vi "10kA Tripping Test.vi"() -> ()   [LabVIEW 2009]
uses:
  Global 6KA.vi
  <vilib>/measure/mamon.llb/Waveform Peak Detection for 1 Chan.vi
  <vilib>/measure/madcrms.llb/Basic Averaged DC-RMS for 1 Chan.vi
  <vilib>/measure/NI_MAPro.lvlib
  <vilib>/Analysis/NI_AALBase.lvlib
panel:
  in  "计算方式选择":bool
  out "状态显示":string
  in  "Peak to RMS":bool
  out "calc led":bool
  out "start led":bool
  in  "Start":bool
  in  "Calculate":bool
  in  "Pulse 50A":enum32{"50A"}(tab)
  in  "50A switch":bool=TRUE
  out "power on time":dbl format="%.1f"
  out "Current":dbl format="%.2f"
  in  "I/V Tab":enum32{"设置", "电流波形显示 ", "电压波形显示"}(tab)
  in  "300V":dbl=1.0 format="%.6g"
  in  "确认":bool
  in  "Current Cal.":dbl[](array[numeric])=[1.0, 1.0, 1.0, 1.0] format="%.6f"
  in  "Save setting":bool
  in  "采样频率":u16=50
  in  "采集时间":i32=500 min=20 max=60000 step=1
  in  "预期试验电流":dbl=50.0
  in  "保存图片":bool
  out "End time":dbl
  out "Start time":dbl
  out "Current Graph":cluster{"Y":dbl[], "Y":dbl[]}[](graph)
  out "voltage graph":cluster{"Y":dbl[], "Y":dbl[]}[](graph)
  in  "Quit":bool
  in  "电流传感器量程":i8(slide)=1 min=1 max=50 step=1 scale=1.0..4.0
  # "D1.25KA 剩余电流测试装置  v1.0"
  # "1250A"
  # "300A"
  # "50A"
  # "10A"
  # "脱扣电流和脱扣时间"
  # "(A)"
  # "(ms)"
  # "手动"
  # "自动"
  # "1-50A"
  # "Other"
  # "采集参数"
  # "计量系数"
  # "10A"
  # "(k/s)"
  # "50A"
  # "300A"
  # "1250A"
  # "(ms)"
  # "(A)"
  # "长沙研诺电气设备有限公司"
  # "请将鼠标移动到界面上任意位置，停留2秒钟后会显示帮助信息!"
  # "长沙研诺电气设备有限公司"
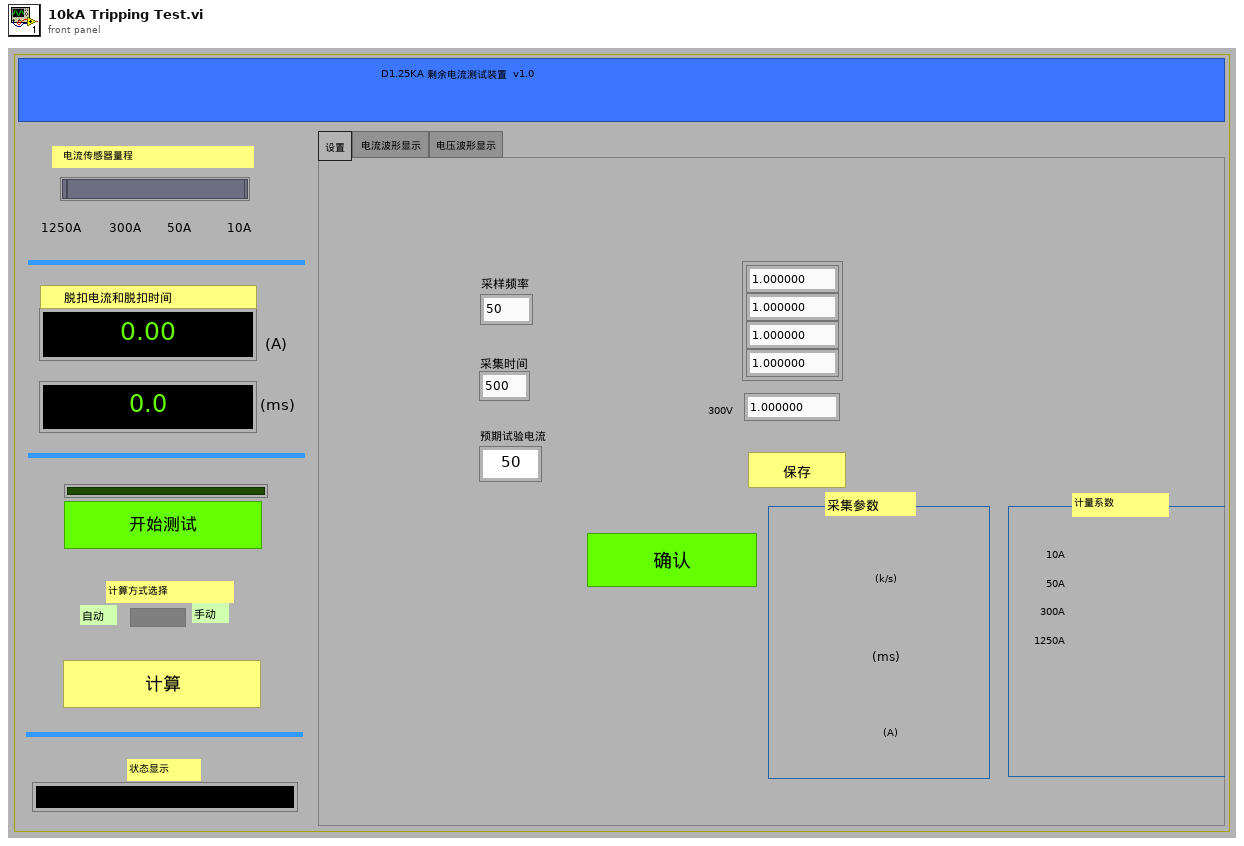
[diagram p1: front panel]
types:
  T1 = enum16{"open", "replace", "create", "open or create", "replace or create", "replace or create with confirmation"}
  T2 = typedef "LVCursorListTypeDef.ctl" = cluster{"Name":string, "Color":u32, "Style":u8, "Point Style":u8, "Name Visible":bool, "Allow Drag":bool, "Cursor Mode":u32, "Plot":i32, "Index":i32, "Position":cluster{"X":dbl, "Y":dbl}, "X Scale":u32, "Y Scale":u32, "Watch Plots":i32[], "Watch All Plots":bool, "Plot Area":i32, "Label Offset":cluster{"X":dbl, "Y":dbl}}[]
  T3 = cluster{"Name":string, "Color":u32, "Style":u8, "Point Style":u8, "Name Visible":bool, "Allow Drag":bool, "Cursor Mode":u32, "Plot":i32, "Index":i32, "Position":cluster{"X":dbl, "Y":dbl}, "X Scale":u32, "Y Scale":u32, "Watch Plots":i32[], "Watch All Plots":bool, "Plot Area":i32, "Label Offset":cluster{"X":dbl, "Y":dbl}}
  T4 = typedef "imagedata.ctl" = cluster{"image type":i32, "image depth":i32, "image":u8[], "mask":u8[], "colors":u32[], "Rectangle":cluster{"left":i16, "top":i16, "right":i16, "bottom":i16}}
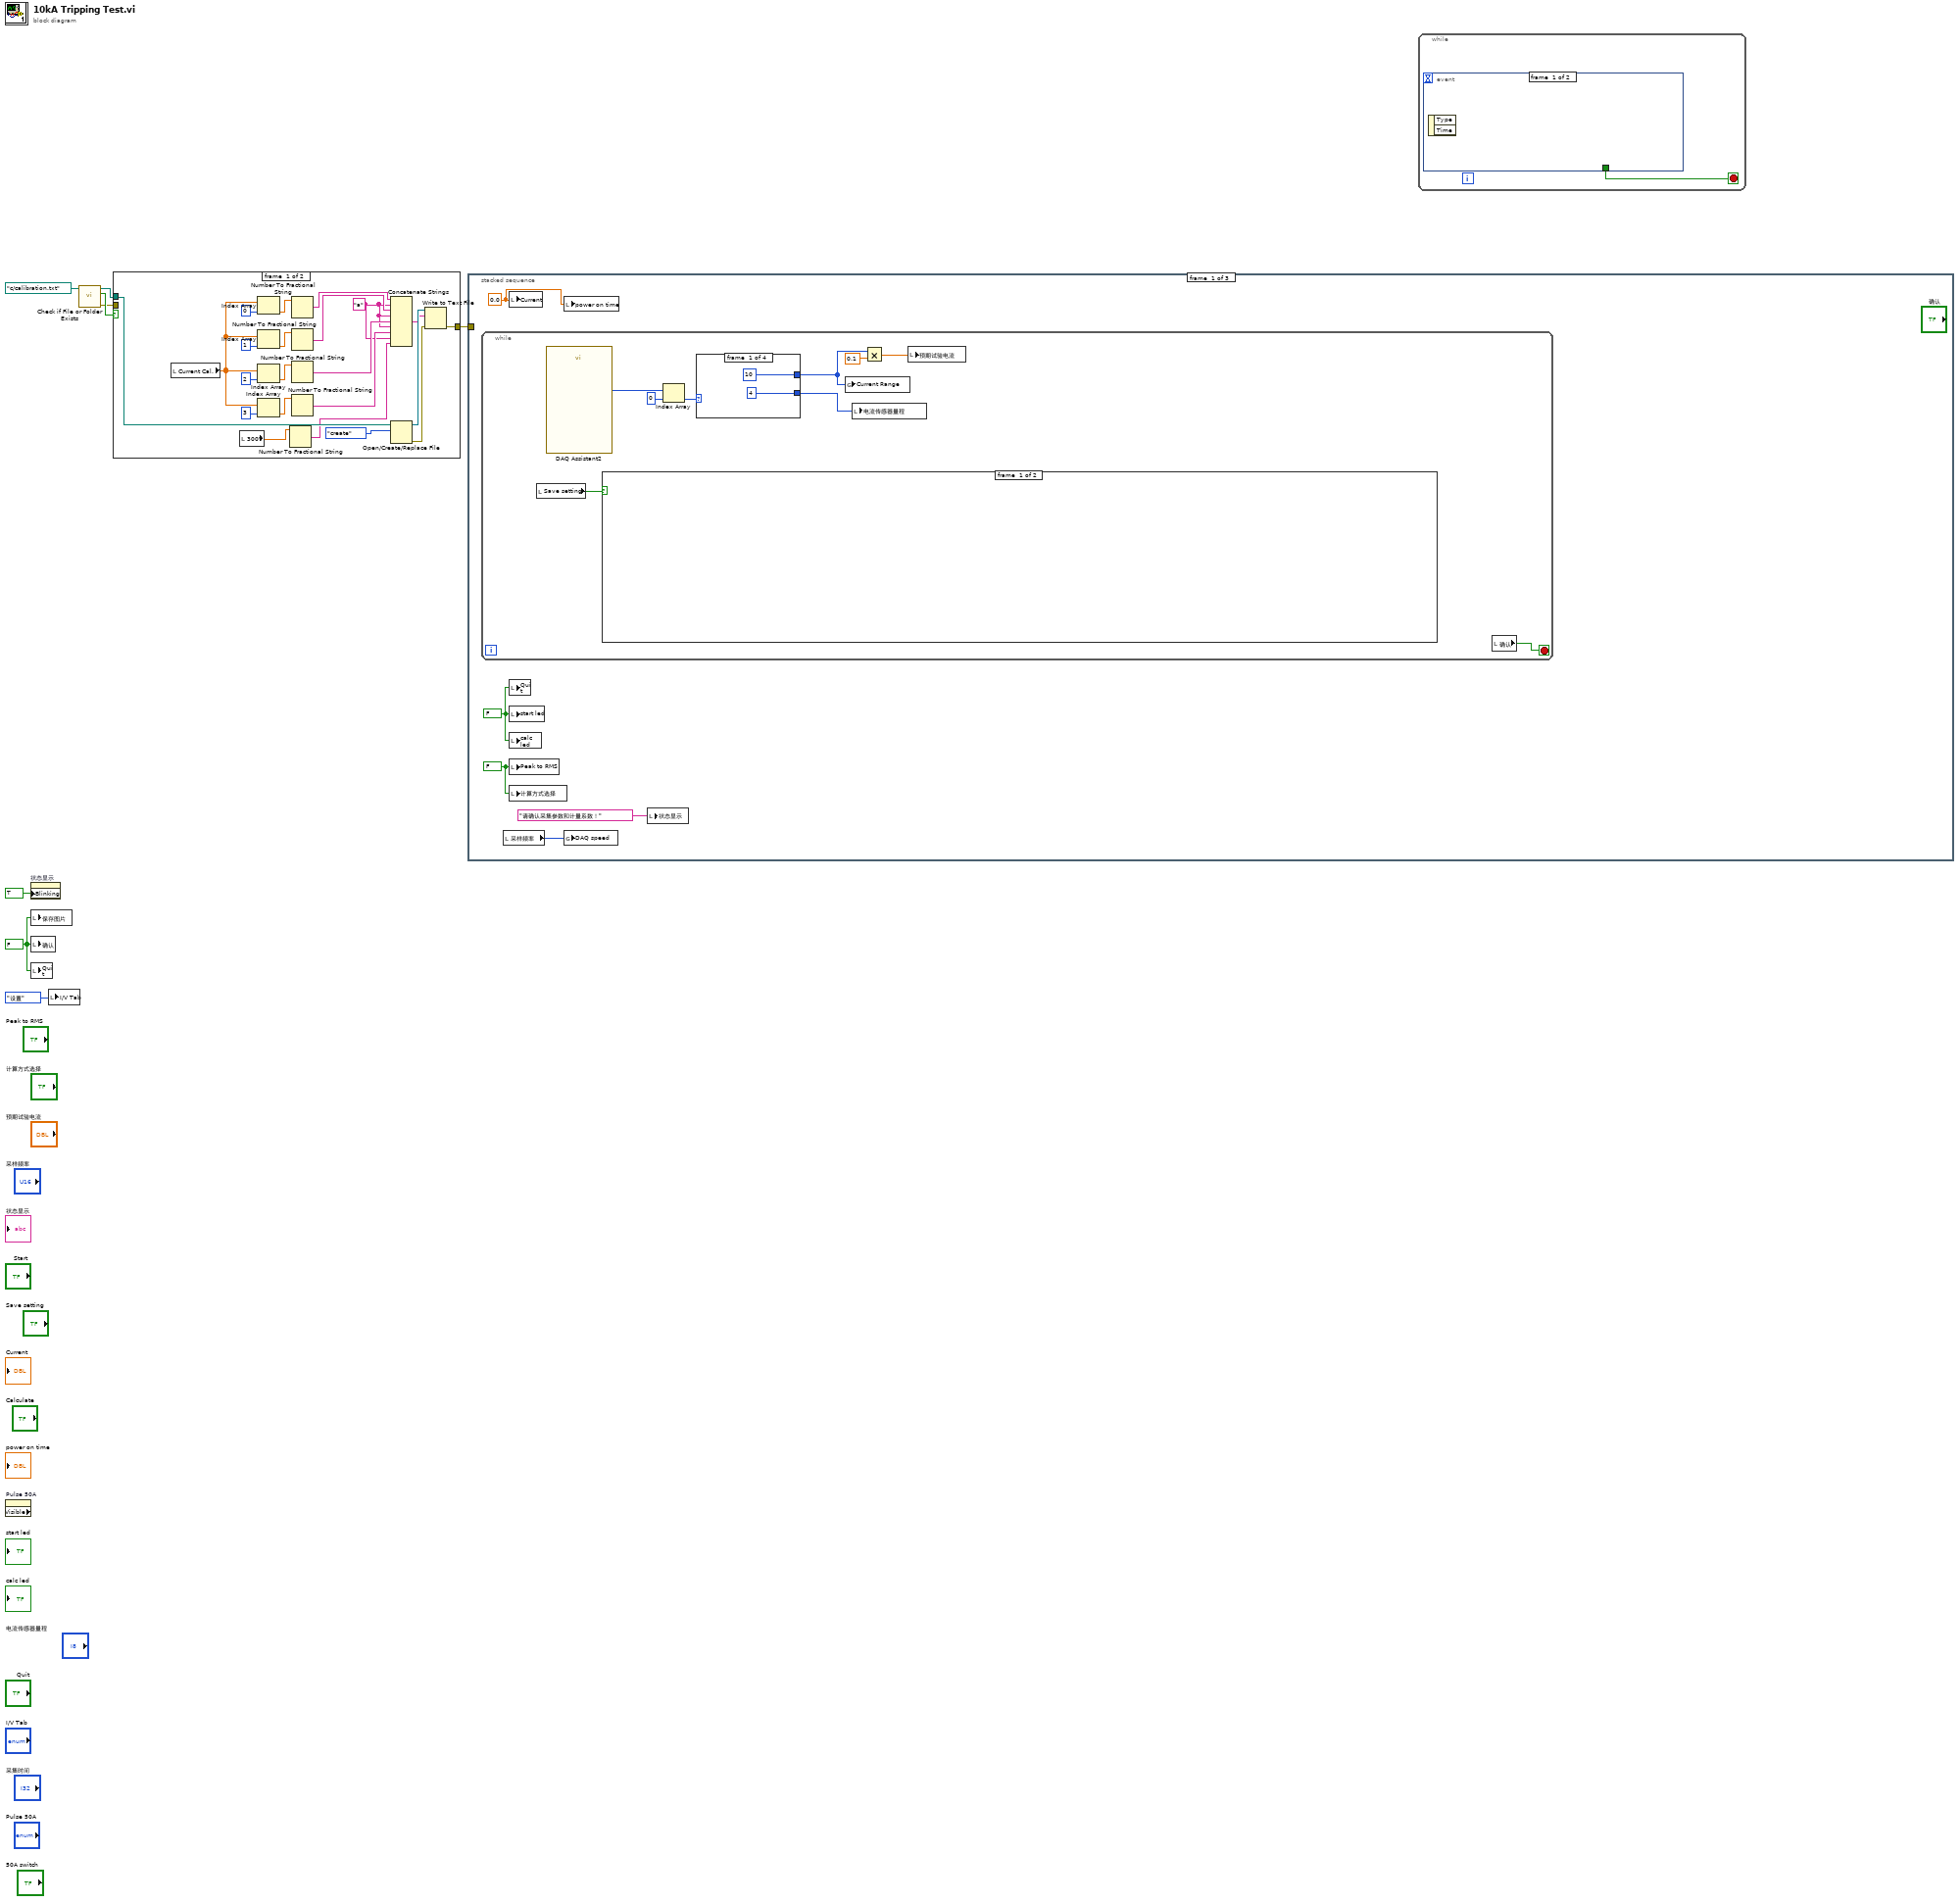
[diagram p0: block diagram]
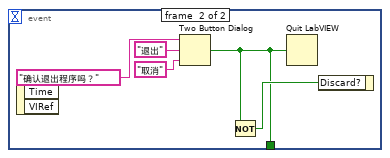
[diagram p2: hidden frame]
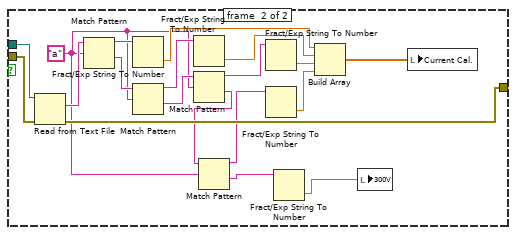
[diagram p3: hidden frame]
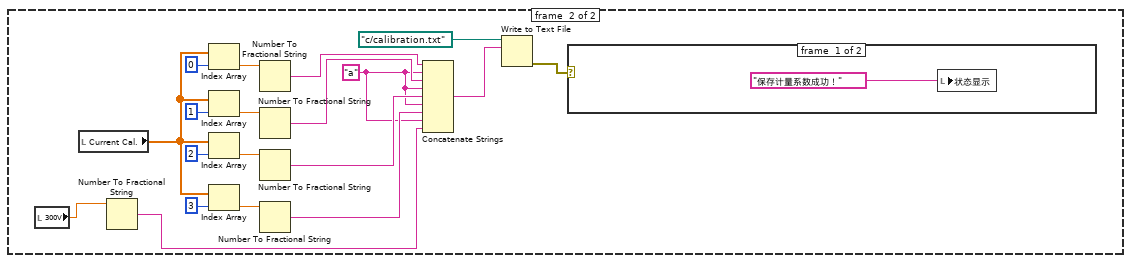
[diagram p4: hidden frame]
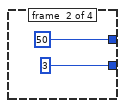
[diagram p6: hidden frame]
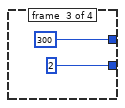
[diagram p7: hidden frame]
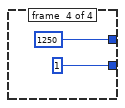
[diagram p8: hidden frame]
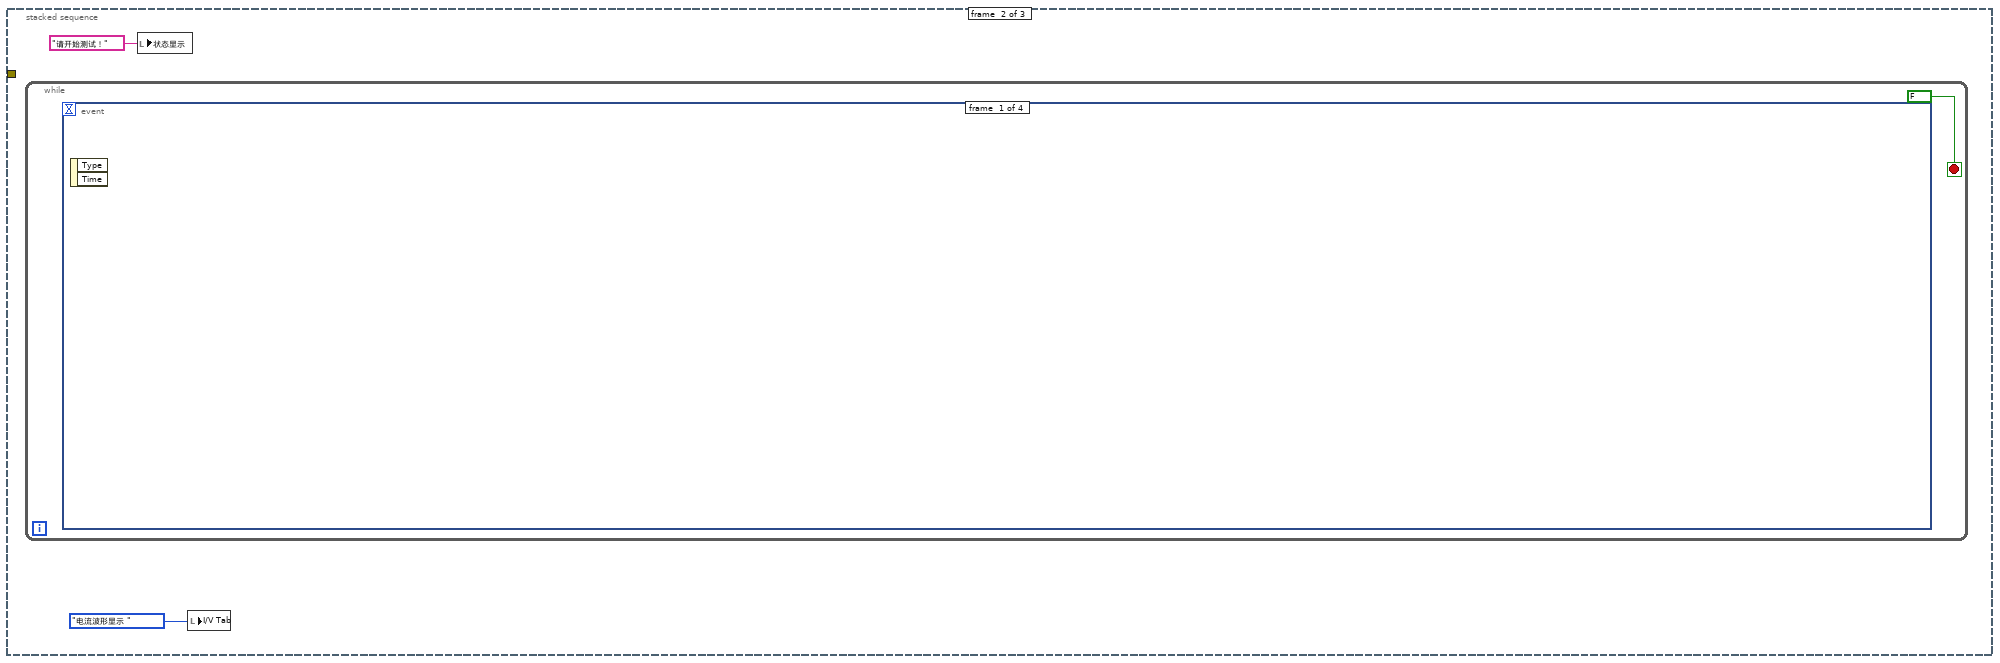
[diagram p9: hidden frame]
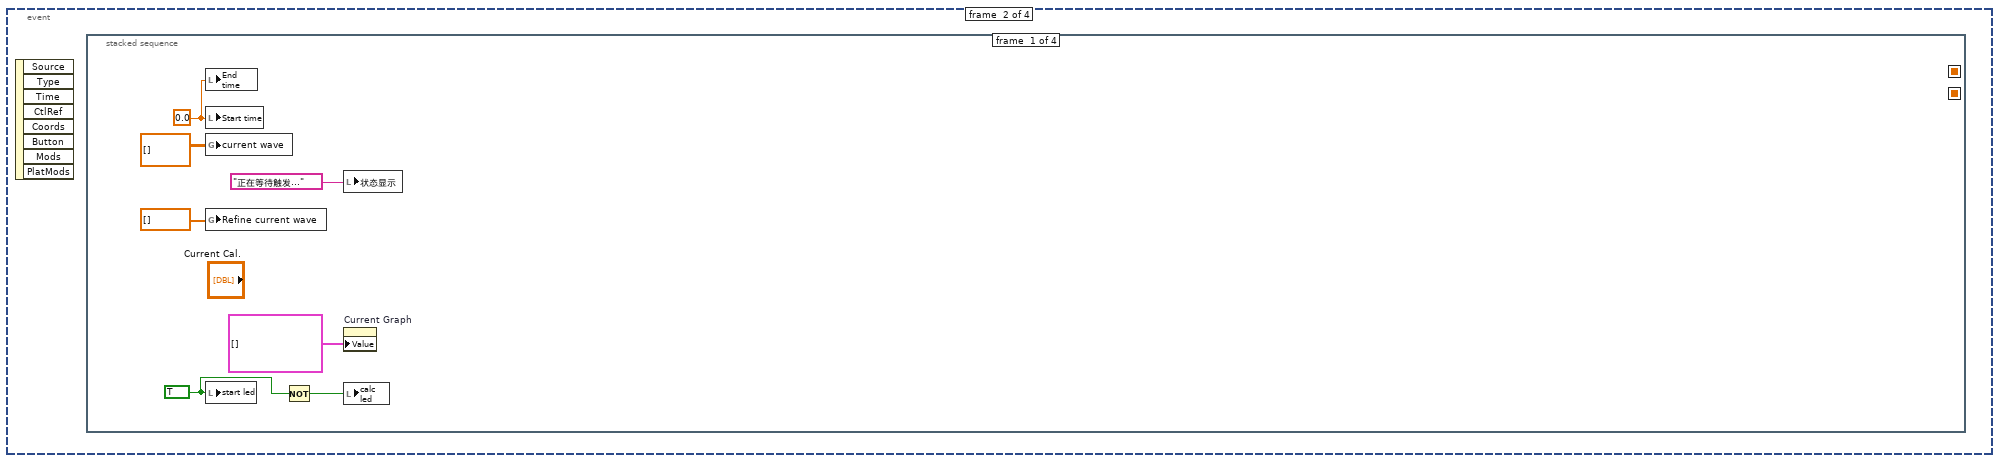
[diagram p10: hidden frame]
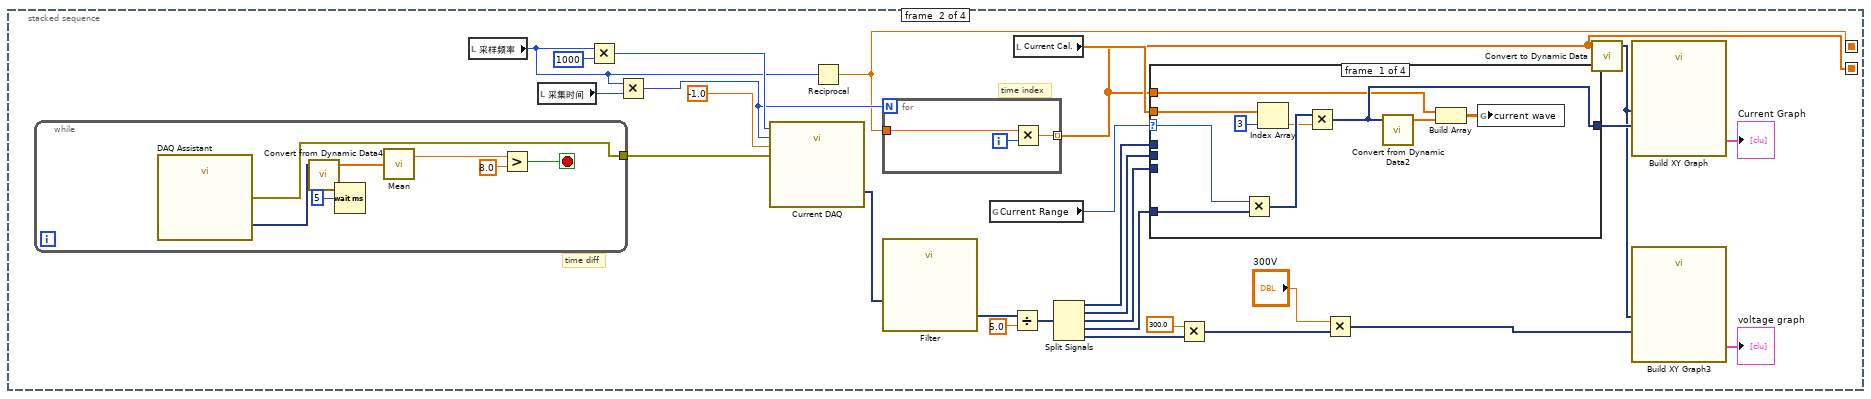
[diagram p11: hidden frame]
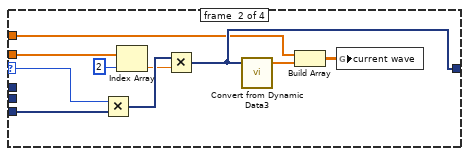
[diagram p12: hidden frame]
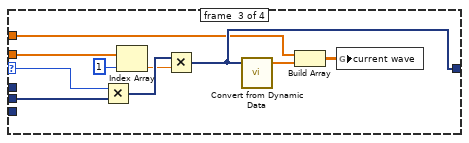
[diagram p13: hidden frame]
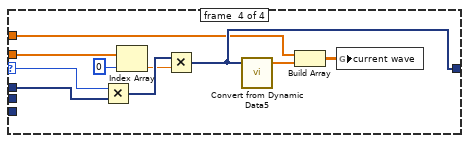
[diagram p14: hidden frame]
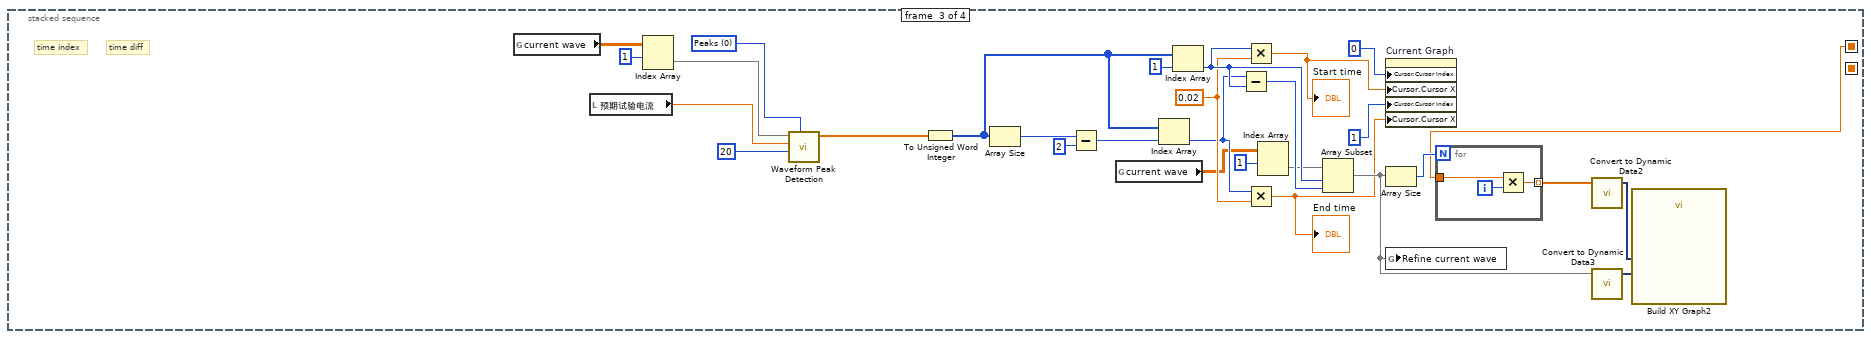
[diagram p15: hidden frame]
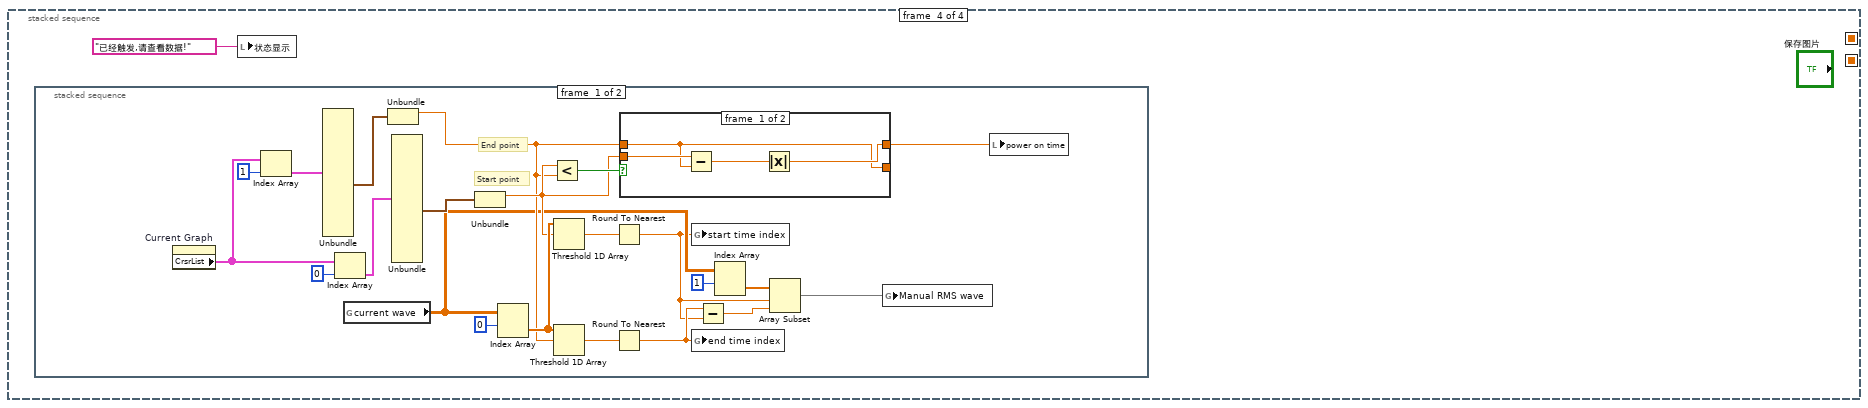
[diagram p16: hidden frame]
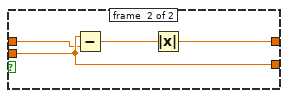
[diagram p17: hidden frame]
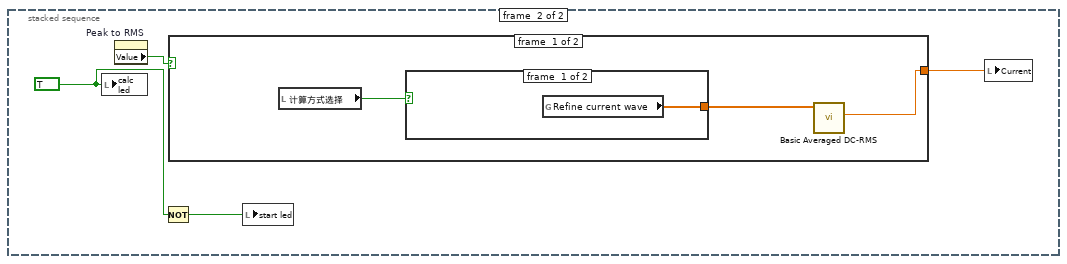
[diagram p18: hidden frame]
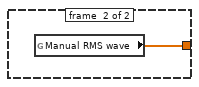
[diagram p19: hidden frame]
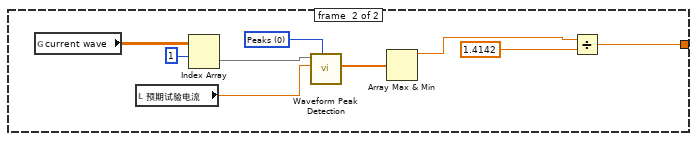
[diagram p20: hidden frame]
diagram:
  w2 = FALSE ("Quit")
  n1 = property on="Pulse 50A" class="TabCtl (strict)" props=["Visible"]() -> ()  [unwired: 2 in, 3 out]
  n2 = property on="状态显示" class="Str"("Blinking"=TRUE) -> ()  [unwired: 2 in, 2 out]
  n3 = local write "保存图片"(w2) -> ()
  n4 = local write "确认"(w2) -> ()
  n5 = local write "Quit"(w2) -> ()
  n6 = local write "I/V Tab"(enum32{"设置", "电流波形显示 "}."设置" ("I/V Tab")) -> ()
  n7 = call <vilib>:"Check if File or Folder Exists.vi"("path"=path "c:/calibration.txt") -> ("error out"=w5:errorcluster, "file or folder exists?"=w7:bool, "dup path"=w4:path)  [unwired: 1 in, 7 out]
  n8 = case shown="False" w7 {
    tunnel: [w16 w47] -> w6
    tunnel: w5 -> [_ w48]
    tunnel: w4 -> [w30 w49]
    frame #0 {
      w11 = "a"
      n9 = local read "Current Cal."() -> (w13:dbl[])
      n10 = local read "300V"() -> (w9:dbl)
      n11 = Index Array(array=w13, index=0) -> (element=w25:dbl)
      n12 = Index Array(array=w13, index=1) -> (element=w22:dbl)
      n13 = Index Array(array=w13, index=2) -> (element=w21:dbl)
      n14 = Index Array(array=w13, index=3) -> (element=w15:dbl)
      n15 = Number To Fractional String(number=w9) -> (F-format string=w10:string)  [unwired: 3 out]
      n16 = Number To Fractional String(number=w25) -> (F-format string=w20:string)  [unwired: 3 out]
      n17 = Number To Fractional String(number=w22) -> (F-format string=w19:string)  [unwired: 3 out]
      n18 = Number To Fractional String(number=w21) -> (F-format string=w18:string)  [unwired: 3 out]
      n19 = Number To Fractional String(number=w15) -> (F-format string=w12:string)  [unwired: 3 out]
      n20 = Concatenate Strings(w20, w11, w19, w11, w18, w11, w12, w11, w10) -> (w17:string)
      n21 = Open/Create/Replace File(file path (use dialog)=w30, operation (0:open)=T1."create") -> (refnum out=w27:refnum<file>, error out=w28:errorcluster)  [unwired: 1 in, 4 out]
      n22 = Write to Text File(file (use dialog)=w27, text=w17, error in=w28) -> (error out=w16:errorcluster)  [unwired: 3 out]
    }
    frame #1 {
      w34 = "a" ("regular expression")
      n23 = Read from Text File(file (use dialog)=w49, error in=w48) -> (text=w46:string, error out=w47:errorcluster)  [unwired: 4 out]
      n24 = Match Pattern(string=w46, regular expression=w34) -> (before substring=w45:string, after substring=w44:string)  [unwired: 3 out]
      n25 = Fract/Exp String To Number(string=w45) -> (number=w42:dbl)  [unwired: 4 out]
      n26 = Match Pattern(string=w44, regular expression=w34) -> (before substring=w43:string, after substring=w38:string)  [unwired: 3 out]
      n27 = Fract/Exp String To Number(string=w43) -> (number=w41:dbl)  [unwired: 4 out]
      n28 = Match Pattern(string=w38, regular expression=w34) -> (before substring=w37:string, after substring=w35:string)  [unwired: 3 out]
      n29 = Match Pattern(string=w35, regular expression=w34) -> (before substring=w33:string, after substring=w32:string)  [unwired: 3 out]
      n30 = Fract/Exp String To Number(string=w37) -> (number=w40:dbl)  [unwired: 4 out]
      n31 = Fract/Exp String To Number(string=w33) -> (number=w36:dbl)  [unwired: 4 out]
      n32 = Fract/Exp String To Number(string=w32) -> (number=w31:dbl)  [unwired: 4 out]
      n33 = Build Array(w42, w41, w40, w36) -> (w39:dbl[])
      n34 = local write "300V"(w31) -> ()
      n35 = local write "Current Cal."(w39) -> ()
    }
  }
  n36 = stacked-sequence {
    tunnel: w6 -> [_ _ _]
    frame #0 {
      w54 = FALSE ("Pulse or full")
      w52 = FALSE ("DAQ Stopped")
      w51 = 0.0 ("A current RMS")
      n37 = while {
        stop <- w59 stop-if-true
        n38 = local read "Save setting"() -> (w58:bool)
        n39 = call "DAQ Assistant2"() -> ("data"=w60:u32[])  [unwired: 3 in, 16 out]
        n40 = case shown="True" w58 {
          frame #0 {
          }
          frame #1 {
            w66 = "a"
            n41 = local read "300V"() -> (w64:dbl)
            n42 = local read "Current Cal."() -> (w68:dbl[])
            n43 = Number To Fractional String(number=w64) -> (F-format string=w65:string)  [unwired: 3 out]
            n44 = Index Array(array=w68, index=0) -> (element=w81:dbl)
            n45 = Index Array(array=w68, index=1) -> (element=w78:dbl)
            n46 = Index Array(array=w68, index=2) -> (element=w77:dbl)
            n47 = Index Array(array=w68, index=3) -> (element=w69:dbl)
            n48 = Number To Fractional String(number=w81) -> (F-format string=w76:string)  [unwired: 3 out]
            n49 = Number To Fractional String(number=w78) -> (F-format string=w75:string)  [unwired: 3 out]
            n50 = Number To Fractional String(number=w77) -> (F-format string=w74:string)  [unwired: 3 out]
            n51 = Number To Fractional String(number=w69) -> (F-format string=w67:string)  [unwired: 3 out]
            n52 = Concatenate Strings(w76, w66, w75, w66, w74, w66, w67, w66, w65) -> (w73:string)
            n53 = Write to Text File(file (use dialog)=path "c:/calibration.txt", text=w73) -> (error out=w71:errorcluster)  [unwired: 1 in, 3 out]
            n54 = case shown="No Error" w71 {
              frame #0 {
                n55 = local write "状态显示"("保存计量系数成功！" ("message")) -> ()
              }
              frame #1 {
              }
            }
          }
        }
        n56 = Index Array(array=w60, index=0) -> (element=w61:u32)
        n57 = case shown="8" w61 {
          tunnel: [10 50 300 1250] -> w57
          tunnel: [4 3 2 1] -> w63
          frame #0 {
          }
          frame #1 {
          }
          frame #2 {
          }
          frame #3 {
          }
        }
        n58 = global write "Global 6KA.vi" "Current Range"(w57) -> ()
        n59 = local write "电流传感器量程"(w63) -> ()
        n60 = Multiply(x=w57, y=0.1) -> (x*y=w55:dbl)
        n61 = local write "预期试验电流"(w55) -> ()
        n62 = local read "确认"() -> (w59:bool)
      }
      n63 = local read "采样频率"() -> (w53:u16)
      n64 = local write "Current"(w51) -> ()
      n65 = local write "Quit"(w54) -> ()
      n66 = local write "start led"(w54) -> ()
      n67 = local write "calc led"(w54) -> ()
      n68 = local write "Peak to RMS"(w52) -> ()
      n69 = local write "计算方式选择"(w52) -> ()
      n70 = local write "power on time"(w51) -> ()
      n71 = global write "Global 6KA.vi" "DAQ speed"(w53) -> ()
      n72 = local write "状态显示"("请确认采集参数和计量系数！" ("状态")) -> ()
    }
    frame #1 {
      n73 = while {
        stop <- FALSE stop-if-true
        n74 = event shown="[3] \"Calculate\": Value Change" {
          selector: _ -> [_ _ _ _]
          dyn-events: _ -> [_ _ _ _]
          timeout: _ -> [_ _ _ _]
          event #0 {
            n75 = event-data() -> ()  [unwired: 3 out]
          }
          event #1 {
            n76 = event-data() -> ()  [unwired: 9 out]
            n77 = stacked-sequence {
              seq-local: [_ w118 _ _] -> [_ _ _ _]
              seq-local: [_ w119 _ _] -> [_ _ w197 _]
              frame #0 {
                w98 = 0.0 ("End time")
                w100 = TRUE ("start led")
                n78 = local write "End time"(w98) -> ()
                n79 = local write "Start time"(w98) -> ()
                n80 = global write "Global 6KA.vi" "current wave"(dbl[][] [] ("current wave")) -> ()
                n81 = global write "Global 6KA.vi" "Refine current wave"(dbl[] [] ("current wave")) -> ()
                n82 = local write "start led"(w100) -> ()
                n83 = Not(x=w100) -> (.not. x?=w101:bool)
                n84 = local write "状态显示"("正在等待触发..." ("状态显示")) -> ()
                n85 = property on="Current Graph" class="XYGraph (strict)"("Value"=cluster{"Y":dbl[], "Y":dbl[]}[] [] ("Current Graph")) -> ()  [unwired: 2 in, 2 out]
                n86 = local write "calc led"(w101) -> ()
              }
              frame #1 {
                # "time diff"
                # "time index"
                n87 = while {
                  tunnel: [w136] -> w116
                  stop <- w134 stop-if-true
                  n88 = call "DAQ Assistant"() -> ("data"=w133:dynamicdata, "error out"=w136:errorcluster)  [unwired: 17 in, 1 out]
                  n89 = call "Convert from Dynamic Data4"("Dynamic Data Type"=w133) -> ("Array"=w132:dbl[])  [unwired: 3 in]
                  n90 = Wait (ms)(milliseconds to wait=u32 5) -> ()  [unwired: 1 out]
                  n91 = call <vilib>:"Mean.vi"("X"=w132) -> ("mean"=w131:dbl)  [unwired: 1 out]
                  n92 = Greater?(x=w131, y=8.0) -> (0:w134:bool)
                }
                n93 = local read "采样频率"() -> (w121:u16)
                n94 = local read "采集时间"() -> (w126:i32)
                n95 = Multiply(x=w121, y=1000) -> (x*y=w122:i32)
                n96 = Multiply(x=w121, y=w126) -> (x*y=w120:i32)
                n97 = call "Current DAQ"("rate"=w122, "number of samples"=w120, "timeout (s)"=-1.0, "error in"=w116) -> ("data"=w117:dynamicdata)  [unwired: 1 in, 14 out]
                n98 = Reciprocal(x=w121) -> (1/x=w119:dbl)
                n99 = for {
                  N: w120 -> [_]
                  tunnel: [w137] -> w118 mode=indexing
                  tunnel: w119 -> [w138]
                  i -> [w139]
                  n100 = Multiply(x=w138, y=w139) -> (x*y=w137:dbl)
                }
                n101 = call "Filter"("Signal"=w117) -> ("Filtered Signal"=w113:dynamicdata)  [unwired: 9 in, 1 out]
                n102 = global read "Global 6KA.vi" "Current Range"() -> (w129:i16)
                n103 = Divide(x=w113, y=5.0) -> (x/y=w114:dynamicdata)
                n104 = local read "Current Cal."() -> (w123:dbl[])
                n105 = Split Signals(w114) -> (w109:dynamicdata, w110:dynamicdata, w111:dynamicdata, w115:dynamicdata, w108:dynamicdata)  [unwired: 5 in]
                n106 = case shown="10" w129 {
                  selector: w129 -> [w149 w159 w169 w179]
                  tunnel: [w143 w154 w164 w174] -> w125
                  tunnel: w123 -> [w145 w156 w166 w176]
                  tunnel: w115 -> [w148 _ _ _]
                  tunnel: w118 -> [w141 w152 w161 w171]
                  tunnel: w111 -> [_ w150 _ _]
                  tunnel: w110 -> [_ _ w160 _]
                  tunnel: w109 -> [_ _ _ w170]
                  frame #0 {
                    n107 = Multiply(x=w149, y=w148) -> (x*y=w147:dynamicdata)
                    n108 = Index Array(array=w145, index=3) -> (element=w144:dbl)
                    n109 = Multiply(x=w147, y=w144) -> (x*y=w143:dynamicdata)
                    n110 = call "Convert from Dynamic Data2"("Dynamic Data Type"=w143) -> ("Array"=w142:dbl[])  [unwired: 3 out]
                    n111 = Build Array(w141, w142) -> (w140:dbl[][])
                    n112 = global write "Global 6KA.vi" "current wave"(w140) -> ()
                  }
                  frame #1 {
                    n113 = Multiply(x=w159, y=w150) -> (x*y=w158:dynamicdata)
                    n114 = Index Array(array=w156, index=2) -> (element=w155:dbl)
                    n115 = Multiply(x=w158, y=w155) -> (x*y=w154:dynamicdata)
                    n116 = call "Convert from Dynamic Data3"("Dynamic Data Type"=w154) -> ("Array"=w153:dbl[])  [unwired: 3 out]
                    n117 = Build Array(w152, w153) -> (w151:dbl[][])
                    n118 = global write "Global 6KA.vi" "current wave"(w151) -> ()
                  }
                  frame #2 {
                    n119 = Multiply(x=w169, y=w160) -> (x*y=w168:dynamicdata)
                    n120 = Index Array(array=w166, index=1) -> (element=w165:dbl)
                    n121 = Multiply(x=w168, y=w165) -> (x*y=w164:dynamicdata)
                    n122 = call "Convert from Dynamic Data"("Dynamic Data Type"=w164) -> ("Array"=w163:dbl[])  [unwired: 3 out]
                    n123 = Build Array(w161, w163) -> (w162:dbl[][])
                    n124 = global write "Global 6KA.vi" "current wave"(w162) -> ()
                  }
                  frame #3 {
                    n125 = Multiply(x=w179, y=w170) -> (x*y=w178:dynamicdata)
                    n126 = Index Array(array=w176, index=0) -> (element=w175:dbl)
                    n127 = Multiply(x=w178, y=w175) -> (x*y=w174:dynamicdata)
                    n128 = call "Convert from Dynamic Data5"("Dynamic Data Type"=w174) -> ("Array"=w173:dbl[])  [unwired: 3 out]
                    n129 = Build Array(w171, w173) -> (w172:dbl[][])
                    n130 = global write "Global 6KA.vi" "current wave"(w172) -> ()
                  }
                }
                n131 = Multiply(x=300.0, y=w108) -> (x*y=w105:dynamicdata)
                n132 = Multiply(x="300V", y=w105) -> (x*y=w103:dynamicdata)
                n133 = call "Convert to Dynamic Data"("Array"=w118) -> ("Dynamic Data Type"=w107:dynamicdata)  [unwired: 3 out]
                n134 = call "Build XY Graph"("Y Input"=w125, "X Input"=w107) -> ("XY Graph"=→"Current Graph":cluster{"Y":dbl[], "Y":dbl[]}[])  [unwired: 3 in, 6 out]
                n135 = call "Build XY Graph3"("Y Input"=w103, "X Input"=w107) -> ("XY Graph"=→"voltage graph":cluster{"Y":dbl[], "Y":dbl[]}[])  [unwired: 3 in, 6 out]
              }
              frame #2 {
                w191 = 0.02 ("y")
                w208 = u16 0 items=["Peaks", "Valleys"] ("peaks/valleys")
                # "time diff"
                # "time index"
                n136 = global read "Global 6KA.vi" "current wave"() -> (w185:dbl[][])
                n137 = local read "预期试验电流"() -> (w207:dbl)
                n138 = Index Array(array=w185, index (row)=1) -> (element=w183:dbl[])  [unwired: 1 in]
                n139 = call-poly <vilib>:"Waveform Peak Detection.vi"("peaks/valleys"=w208, "width"=20, "threshold"=w207, "Signal In"=w183) -> ("Locations"=w202:dbl[])  [unwired: 3 in, 4 out]
                n140 = To Unsigned Word Integer(number=w202) -> (unsigned 16bit integer=w200:u16[])
                n141 = Array Size(array=w200) -> (size(s)=w204:i32)
                n142 = Subtract(x=w204, y=2) -> (x-y=w201:i32)
                n143 = global read "Global 6KA.vi" "current wave"() -> (w181:dbl[][])
                n144 = Index Array(array=w200, index=w201) -> (element=w190:u16)
                n145 = Index Array(array=w200, index=1) -> (element=w192:u16)
                n146 = Subtract(x=w190, y=w192) -> (x-y=w199:u16)
                n147 = Multiply(x=w192, y=w191) -> (x*y=w187:dbl)
                "Start time" <- w187
                n148 = Multiply(x=w190, y=w191) -> (x*y=w186:dbl)
                "End time" <- w186
                n149 = Index Array(array=w181, index (row)=1) -> (element=w180:dbl[])  [unwired: 1 in]
                n150 = Array Subset(array=w180, index=w192, length=w199) -> (w193:dbl[])
                n151 = property on="Current Graph" class="XYGraph (strict)"("Cursor.Cursor Index"=0, "Cursor.Cursor X"=w187, "Cursor.Cursor Index"=1, "Cursor.Cursor X"=w186) -> ()  [unwired: 2 in, 2 out]
                n152 = Array Size(array=w193) -> (size(s)=w198:i32)
                n153 = global write "Global 6KA.vi" "Refine current wave"(w193) -> ()
                n154 = for {
                  N: w198 -> [_]
                  tunnel: w197 -> [w210]
                  tunnel: [w209] -> w196 mode=indexing
                  i -> [w211]
                  n155 = Multiply(x=w210, y=w211) -> (x*y=w209:dbl)
                }
                n156 = call "Convert to Dynamic Data2"("Array"=w196) -> ("Dynamic Data Type"=w195:dynamicdata)  [unwired: 3 out]
                n157 = call "Convert to Dynamic Data3"("Array"=w193) -> ("Dynamic Data Type"=w194:dynamicdata)  [unwired: 3 out]
                n158 = call "Build XY Graph2"("Y Input"=w194, "X Input"=w195) -> ()  [unwired: 3 in, 7 out]
              }
              frame #3 {
                n159 = stacked-sequence {
                  frame #0 {
                    # "End point"
                    # "Start point"
                    n160 = property on="Current Graph" class="XYGraph (strict)"() -> ("CrsrList"=w227:T2)  [unwired: 2 in, 2 out]
                    n161 = Index Array(array=w227, index=1) -> (element=w232:T3)
                    n162 = Unbundle(w232) -> ("Position"=w233:cluster{"X":dbl, "Y":dbl})  [unwired: 15 out]
                    n163 = Index Array(array=w227, index=0) -> (element=w230:T3)
                    n164 = global read "Global 6KA.vi" "current wave"() -> (w221:dbl[][])
                    n165 = Unbundle(w233) -> ("X"=w222:dbl)  [unwired: 1 out]
                    n166 = Unbundle(w230) -> ("Position"=w231:cluster{"X":dbl, "Y":dbl})  [unwired: 15 out]
                    n167 = Unbundle(w231) -> ("X"=w223:dbl)  [unwired: 1 out]
                    n168 = Index Array(array=w221, index (row)=0) -> (element=w224:dbl[])  [unwired: 1 in]
                    n169 = Less?(x=w223, y=w222) -> (x < y?=w234:bool)
                    n170 = Threshold 1D Array(2:w223, 3:w224) -> (0:w219:dbl)  [unwired: 1 out]
                    n171 = Threshold 1D Array(2:w222, 3:w224) -> (0:w218:dbl)  [unwired: 1 out]
                    n172 = Round To Nearest(number=w219) -> (nearest integer value=w215:dbl)
                    n173 = Round To Nearest(number=w218) -> (nearest integer value=w216:dbl)
                    n174 = case shown="True" w234 {
                      tunnel: w222 -> [w235 w239]
                      tunnel: w223 -> [w236 w240]
                      tunnel: [w235 w240] -> _
                      tunnel: [w238 w241] -> w226
                      frame #0 {
                        n175 = Subtract(x=w236, y=w235) -> (x-y=w237:dbl)
                        n176 = Absolute Value(x=w237) -> (abs(x)=w238:dbl)
                      }
                      frame #1 {
                        n177 = Subtract(x=w240, y=w239) -> (x-y=w242:dbl)
                        n178 = Absolute Value(x=w242) -> (abs(x)=w241:dbl)
                      }
                    }
                    n179 = global write "Global 6KA.vi" "start time index"(w215) -> ()
                    n180 = global write "Global 6KA.vi" "end time index"(w216) -> ()
                    n181 = Subtract(x=w216, y=w215) -> (x-y=w214:dbl)
                    n182 = Index Array(array=w221, index (row)=1) -> (element=w217:dbl[])  [unwired: 1 in]
                    n183 = Array Subset(array=w217, index=w215, length=w214) -> (w213:dbl[])
                    n184 = global write "Global 6KA.vi" "Manual RMS wave"(w213) -> ()
                    n185 = local write "power on time"(w226) -> ()
                  }
                  frame #1 {
                    w245 = TRUE ("calc led")
                    n186 = local write "calc led"(w245) -> ()
                    n187 = property on="Peak to RMS" class="Bool (strict)"() -> ("Value"=w243:bool)  [unwired: 2 in, 2 out]
                    n188 = Not(x=w245) -> (.not. x?=w246:bool)
                    n189 = case shown="False" w243 {
                      tunnel: [w248 w256] -> w244
                      frame #0 {
                        n190 = local read "计算方式选择"() -> (w247:bool)
                        n191 = case shown="False" w247 {
                          tunnel: [w250 w251] -> w249
                          frame #0 {
                            n192 = global read "Global 6KA.vi" "Refine current wave"() -> (w250:dbl[])
                          }
                          frame #1 {
                            n193 = global read "Global 6KA.vi" "Manual RMS wave"() -> (w251:dbl[])
                          }
                        }
                        n194 = call-poly <vilib>:"Basic Averaged DC-RMS.vi"("signal in"=w249) -> ("RMS value"=w248:dbl)  [unwired: 4 in, 6 out]
                      }
                      frame #1 {
                        w260 = u16 0 items=["Peaks", "Valleys"] ("peaks/valleys")
                        n195 = global read "Global 6KA.vi" "current wave"() -> (w254:dbl[][])
                        n196 = local read "预期试验电流"() -> (w255:dbl)
                        n197 = Index Array(array=w254, index (row)=1) -> (element=w252:dbl[])  [unwired: 1 in]
                        n198 = call-poly <vilib>:"Waveform Peak Detection.vi"("peaks/valleys"=w260, "threshold"=w255, "Signal In"=w252) -> ("Amplitudes"=w259:dbl[])  [unwired: 4 in, 4 out]
                        n199 = Array Max & Min(array=w259) -> (max value=w258:dbl)  [unwired: 3 out]
                        n200 = Divide(x=w258, y=1.4142) -> (x/y=w256:dbl)
                      }
                    }
                    n201 = local write "start led"(w246) -> ()
                    n202 = local write "Current"(w244) -> ()
                  }
                }
                n203 = local write "状态显示"("已经触发,请查看数据!" ("状态显示")) -> ()
              }
            }
          }
          event #2 {
            n204 = event-data() -> ()  [unwired: 7 out]
            n205 = local write "保存图片"(FALSE ("保存图片")) -> ()
            n206 = invoke class="VI" method="FP.Get Image"() -> ("image data"=w262:T4)  [unwired: 6 in, 5 out]
            n207 = local write "状态显示"("图片保存成功!" ("状态显示")) -> ()
            n208 = call <vilib>:"Write PNG File.vi"("image data"=w262) -> ()  [unwired: 2 in, 9 out]
          }
          event #3 {
            n209 = event-data() -> ()  [unwired: 7 out]
            n210 = stacked-sequence {
              frame #0 {
                # "End point"
                # "Start point"
                n211 = property on="Current Graph" class="XYGraph (strict)"() -> ("CrsrList"=w278:T2)  [unwired: 2 in, 2 out]
                n212 = Index Array(array=w278, index=1) -> (element=w283:T3)
                n213 = Unbundle(w283) -> ("Position"=w284:cluster{"X":dbl, "Y":dbl})  [unwired: 15 out]
                n214 = Index Array(array=w278, index=0) -> (element=w281:T3)
                n215 = global read "Global 6KA.vi" "current wave"() -> (w272:dbl[][])
                n216 = Unbundle(w284) -> ("X"=w273:dbl)  [unwired: 1 out]
                n217 = Unbundle(w281) -> ("Position"=w282:cluster{"X":dbl, "Y":dbl})  [unwired: 15 out]
                n218 = Unbundle(w282) -> ("X"=w274:dbl)  [unwired: 1 out]
                n219 = Index Array(array=w272, index (row)=0) -> (element=w275:dbl[])  [unwired: 1 in]
                n220 = Less?(x=w274, y=w273) -> (x < y?=w285:bool)
                n221 = Threshold 1D Array(2:w274, 3:w275) -> (0:w270:dbl)  [unwired: 1 out]
                n222 = Threshold 1D Array(2:w273, 3:w275) -> (0:w269:dbl)  [unwired: 1 out]
                n223 = Round To Nearest(number=w270) -> (nearest integer value=w266:dbl)
                n224 = Round To Nearest(number=w269) -> (nearest integer value=w267:dbl)
                n225 = case shown="True" w285 {
                  tunnel: w273 -> [w286 w290]
                  tunnel: w274 -> [w287 w291]
                  tunnel: [w286 w291] -> _
                  tunnel: [w289 w292] -> w277
                  frame #0 {
                    n226 = Subtract(x=w287, y=w286) -> (x-y=w288:dbl)
                    n227 = Absolute Value(x=w288) -> (abs(x)=w289:dbl)
                  }
                  frame #1 {
                    n228 = Subtract(x=w291, y=w290) -> (x-y=w293:dbl)
                    n229 = Absolute Value(x=w293) -> (abs(x)=w292:dbl)
                  }
                }
                n230 = global write "Global 6KA.vi" "start time index"(w266) -> ()
                n231 = global write "Global 6KA.vi" "end time index"(w267) -> ()
                n232 = Subtract(x=w267, y=w266) -> (x-y=w265:dbl)
                n233 = Index Array(array=w272, index (row)=1) -> (element=w268:dbl[])  [unwired: 1 in]
                n234 = Array Subset(array=w268, index=w266, length=w265) -> (w264:dbl[])
                n235 = global write "Global 6KA.vi" "Manual RMS wave"(w264) -> ()
                n236 = local write "power on time"(w277) -> ()
              }
              frame #1 {
                w296 = TRUE ("calc led")
                n237 = local write "calc led"(w296) -> ()
                n238 = property on="Peak to RMS" class="Bool (strict)"() -> ("Value"=w294:bool)  [unwired: 2 in, 2 out]
                n239 = Not(x=w296) -> (.not. x?=w297:bool)
                n240 = case shown="False" w294 {
                  tunnel: [w299 w307] -> w295
                  frame #0 {
                    n241 = local read "计算方式选择"() -> (w298:bool)
                    n242 = case shown="True" w298 {
                      tunnel: [w301 w302] -> w300
                      frame #0 {
                        n243 = global read "Global 6KA.vi" "Refine current wave"() -> (w301:dbl[])
                      }
                      frame #1 {
                        n244 = global read "Global 6KA.vi" "Manual RMS wave"() -> (w302:dbl[])
                      }
                    }
                    n245 = call-poly <vilib>:"Basic Averaged DC-RMS.vi"("signal in"=w300) -> ("RMS value"=w299:dbl)  [unwired: 4 in, 6 out]
                  }
                  frame #1 {
                    w311 = u16 0 items=["Peaks", "Valleys"] ("peaks/valleys")
                    n246 = global read "Global 6KA.vi" "current wave"() -> (w305:dbl[][])
                    n247 = local read "预期试验电流"() -> (w306:dbl)
                    n248 = Index Array(array=w305, index (row)=1) -> (element=w303:dbl[])  [unwired: 1 in]
                    n249 = call-poly <vilib>:"Waveform Peak Detection.vi"("peaks/valleys"=w311, "threshold"=w306, "Signal In"=w303) -> ("Amplitudes"=w310:dbl[])  [unwired: 4 in, 4 out]
                    n250 = Array Max & Min(array=w310) -> (max value=w309:dbl)  [unwired: 3 out]
                    n251 = Divide(x=w309, y=1.4142) -> (x/y=w307:dbl)
                  }
                }
                n252 = local write "start led"(w297) -> ()
                n253 = local write "Current"(w295) -> ()
              }
            }
          }
        }
      }
      n254 = local write "状态显示"("请开始测试！" ("状态显示")) -> ()
      n255 = local write "I/V Tab"(enum32{"设置", "电流波形显示 "}."电流波形显示 " ("I/V Tab")) -> ()
    }
    frame #2 {
      w312 = FALSE ("start led")
      n256 = local write "start led"(w312) -> ()
      n257 = local write "calc led"(w312) -> ()
    }
  }
  n258 = while {
    stop <- w313 stop-if-true
    n259 = event shown="[1] Panel Close?" {
      selector: _ -> [_ _]
      dyn-events: _ -> [_ _]
      timeout: _ -> [_ _]
      tunnel: [_ w314] -> w313
      event #0 {
        n260 = event-data() -> ()  [unwired: 1 in, 2 out]
      }
      event #1 {
        n261 = event-data() -> ()  [unwired: 1 in, 3 out]
        n262 = Two Button Dialog(message="确认退出程序吗？", 1:"取消" ("F button name (\"Cancel\")"), 2:"退出" ("T button name (\"OK\")")) -> (T button?=w314:bool)
        n263 = Not(x=w314) -> (.not. x?=w315:bool)
        n264 = Quit LabVIEW(quit? (T)=w314) -> ()
        n265 = event-data("Discard?"=w315) -> ()  [unwired: 1 in, 1 out]
      }
    }
  }
